vi "ACT_OPEN.vi"(7 "Needle Valve Data.StateValveModbus":T1=enum."OPENING", 8 "error in (no error)":errorcluster, 11 "NeedleValve in":refnum<class "NeedleValve.lvclass">) -> (0 "error out":errorcluster, 3 "NeedleValve out":refnum<class "NeedleValve.lvclass">)   [LabVIEW 2019, in "NeedleValve.lvclass"]
uses:
  NeedleValve.lvclass
  TypeDef/Needle Valve State.ctl
  NeedleValve.lvclass/NeedleValve.ctl
  modbus engine custom/MB_ENGINE_class/cmd enum.ctl
  94d36c57-f1ac-421d-b00d-9da3bb483256.vi
  58a27c99-353e-4e07-9e05-55f5defa50a0.vi
  5313a345-1a18-4309-8791-272529e982b0.vi
  a8bd57a2-6632-4a90-972e-cb7ef7401f3e.vi
  modbus engine custom/MB_ENGINE_class/MB_ENGINE.lvclass
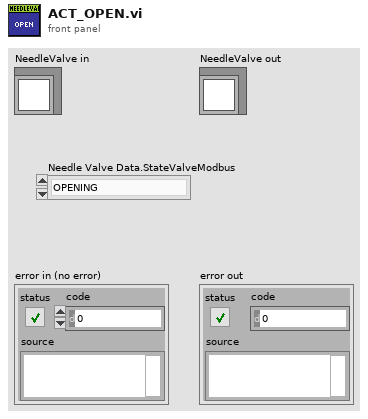
[diagram p1: front panel]
types:
  T1 = typedef "Needle Valve State.ctl" = enum16{"STOPED", "CLOSED", "OPENED", "OPENING", "CLOSING", "FULL_CLOSE", "PREP_OPEN"}
  T2 = typedef "Needle Valve Data.ctl" = cluster{"Engine State":T3, "StateValveModbus":T1, "Alarms":T4, "RAW":i32, "Angele":dbl, "Step":i32, "Encoder":i32, "Kinematic":T5, "Limits":T6, "EncoderMax":i32, "Counter Max Dont Update":i32, "EncoderMin":i32, "Counter Min Dont Update":i32, "Prepere Counter":i32, "STEP INIT":i32, "offset - Angel":dbl}
  T3 = typedef "MB_ENGINE.lvclass/Engine State.ctl" = u16
  T4 = typedef "MB_ENGINE.lvclass/Engine Alarms.ctl" = cluster{"OL":bool, "TF":bool, "STL":bool, "OCP":bool, "CPUV":bool, "UVLO":bool, "SPI_ERROR":bool, "Fault":bool, "OL 2":bool, "TF 2":bool, "STL 2":bool, "OCP 2":bool, "CPUV 2":bool, "UVLO 2":bool, "reserved":bool, "InitDone":bool}
  T5 = typedef "MB_ENGINE.lvclass/Settings.ctl" = cluster{"ACC Steps Per Sec^2":u16, "DEC Steps Per Sec^2":u16, "Min Velosity Step Per Sec":u16, "Max Velosity Step Per Sec":u16, "MicroStep":u16}
  T6 = typedef "MB_ENGINE.lvclass/Limits Status.ctl" = cluster{"Fault 2 Switch":bool, "Fault 1 Switch":bool, "Center(Home)":bool, "Lower Limit":bool, "Upper Limit":bool}
  T7 = typedef "MB_ENGINE.lvclass/cmd enum.ctl" = u16
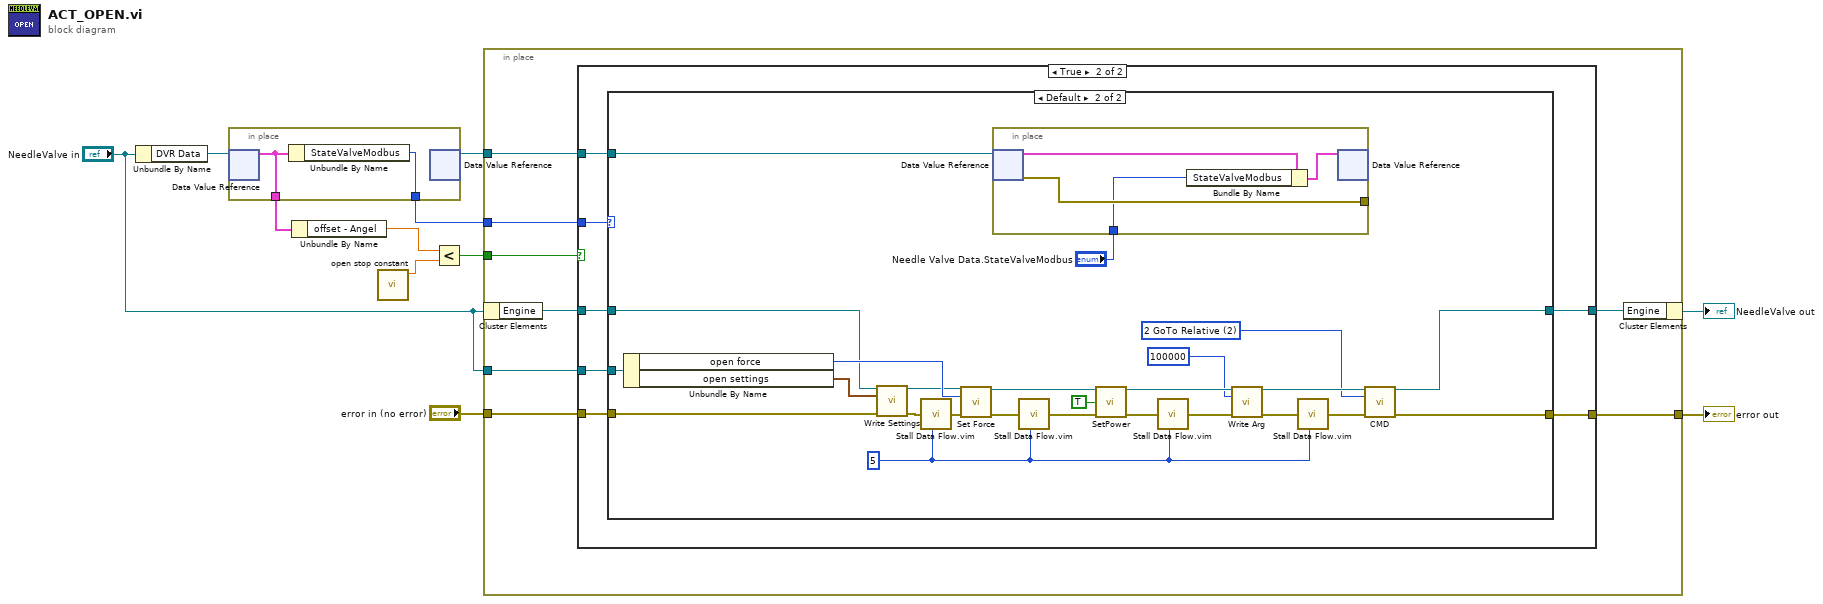
[diagram p0: block diagram]
diagram:
  n1 = Unbundle By Name("NeedleValve in") -> ("DVR Data"=w8:refnum<data-value>)
  n2 = in-place {
    in-place-border: [w13] -> w6
    in-place-border: [w12] -> w3
    n3 = in-place-dvr #1(w8) -> (w12:T2)  [unwired: 1 out]
    n4 = Unbundle By Name(w12) -> ("StateValveModbus"=w13:T1)
    n5 = in-place-dvr #1() -> (w5:refnum<data-value>)  [unwired: 1 in, 1 out]
  }
  n6 = Unbundle By Name(w3) -> ("offset - Angel"=w2:dbl)
  n7 = call "open stop constant.vi"() -> ("angle"=w4:dbl)  [unwired: 11 in]
  n8 = Less?(x=w2, y=w4) -> (x < y?=w1:bool)
  n9 = in-place {
    in-place-border: "NeedleValve in" -> [w21]
    in-place-border: "error in (no error)" -> [w20]
    in-place-border: [w17] -> w10
    in-place-border: w6 -> [w16]
    in-place-border: w5 -> [w15]
    in-place-border: w1 -> [w14]
    n10 = in-place-cluster #2("NeedleValve in") -> ("Engine"=w19:refnum<class "MB_ENGINE.lvclass">)
    n11 = case shown="True" w14 {
      tunnel: w21 -> [_ w30]
      tunnel: w20 -> [w22 w29]
      tunnel: w19 -> [w23 w28]
      tunnel: [w23 w27] -> w18
      tunnel: [w22 w26] -> w17
      tunnel: w16 -> [_ w25]
      tunnel: w15 -> [_ w24]
      frame False {
      }
      frame True {
        n12 = case shown="Default" w25 {
          tunnel: w30 -> [_ w54]
          tunnel: w29 -> [w31 w53]
          tunnel: w28 -> [w32 w52]
          tunnel: [w32 w40] -> w27
          tunnel: [w31 w39] -> w26
          tunnel: w24 -> [_ w34]
          frame "OPENING" {
          }
          frame Default {
            w44 = T7 2 items=["0 Idle"=0, "1 GoTo Absolute Position"=1, "2 GoTo Relative"=2, "10 GoTo Home Position"=10, "11 Set Home Position"=11, "12 Set FindHome Mode"=12, "13 Reset FindHome Mode"=13, "14 Get FindHome State"=14, "20 Hard Stop"=20, "21 HiZ Stop"=21, "22 Soft Stop"=22, "30 Clear Fault"=30, "40 Encoder Set Home"=40, "70 Driver Init"=70] ("cmd to write")
            w35 = u32 5 ("milliseconds to wait")
            n13 = Unbundle By Name(w54) -> ("open force"=w56:u16, "open settings"=w55:T5)
            n14 = call "Write Settings.vi"("class data in"=w52, "cluster"=w55, "error in (no error)"=w53) -> ("class data out"=w51:refnum<class "MB_ENGINE.lvclass">, "error out"=w37:errorcluster)  [unwired: 11 in]
            n15 = call "Stall Data Flow.vim"("value in"=w37, "milliseconds to wait"=w35) -> ("value out"=w36:errorcluster)  [unwired: 1 out]
            n16 = call "Set Force.vi"("class data in"=w51, "percent"=w56, "error in (no error)"=w36) -> ("class data out"=w50:refnum<class "MB_ENGINE.lvclass">, "error out"=w49:errorcluster)  [unwired: 11 in]
            n17 = in-place {
              in-place-border: [w59] -> _
              in-place-border: "Needle Valve Data.StateValveModbus" -> [w58]
              n18 = in-place-dvr #3(w34) -> (w61:T2, w59:errorcluster)
              n19 = Bundle By Name(cluster=w61, "StateValveModbus"=w58) -> (w60:T2)
              n20 = in-place-dvr #3(w60) -> ()  [unwired: 2 out]
            }
            n21 = call "Stall Data Flow.vim"("value in"=w49, "milliseconds to wait"=w35) -> ("value out"=w48:errorcluster)  [unwired: 1 out]
            n22 = call "SetPower.vi"("class data in"=w50, "On"=TRUE, "error in (no error)"=w48) -> ("class data out"=w41:refnum<class "MB_ENGINE.lvclass">, "error out"=w43:errorcluster)  [unwired: 11 in]
            n23 = call "Stall Data Flow.vim"("value in"=w43, "milliseconds to wait"=w35) -> ("value out"=w42:errorcluster)  [unwired: 1 out]
            n24 = call "Write Arg.vi"("class data in"=w41, "ARG U32"=100000, "error in (no error)"=w42) -> ("class data out"=w45:refnum<class "MB_ENGINE.lvclass">, "error out"=w46:errorcluster)  [unwired: 11 in]
            n25 = call "Stall Data Flow.vim"("value in"=w46, "milliseconds to wait"=w35) -> ("value out"=w47:errorcluster)  [unwired: 1 out]
            n26 = call "CMD.vi"("class data in"=w45, "cmd to write"=w44, "error in (no error)"=w47) -> ("class data out"=w40:refnum<class "MB_ENGINE.lvclass">, "error out"=w39:errorcluster)  [unwired: 11 in]
          }
        }
      }
    }
    n27 = in-place-cluster #2("Engine"=w18) -> (→"NeedleValve out":refnum<class "NeedleValve.lvclass">)
  }
  "error out" <- w10
